vi "Do_ADAM_channel.vi"(4 "Scan Period":dbl format="%.2f", 5 "Previous Scan Value":dbl format="%.2f", 6 "Present scan array":dbl[](array[numeric]) format="%.2f", 7 "Value to Output":dbl format="%.2f", 8 "Ch Description":T1 {"Duty" format="%.0b"; "D" format="%#_5g"; "C" format="%#_5g"; "B" format="%#_5g"; "A" format="%#_5g"}, 9 "Ch names":string[](array[string])) -> (0 "Scan comment":string, 1 "Output":dbl format="%.3f")   [LabVIEW 2011]
uses:
  ADAM Client/Sub VIs/ADAM Controls/Ch_description_ADAM.ctl
  ADAM Client/Sub VIs/ADAM Controls/Module_type_ADAM.ctl
  ADAM Client/Sub VIs/ADAM Controls/Function_ADAM.ctl
  ADAM Client/Sub VIs/ADAM Controls/Channel_State.ctl
  ADAM Client/Sub VIs/ADAM Controls/Calib_type_ADAM.ctl
  ADAM Client/Sub VIs/ADAM Controls/Address.ctl
  ADAM Client/Sub VIs/ADAM Controls/Remember_value_mode.ctl
  ADAM Client/Sub VIs/ADAM Controls/Search_mode.ctl
  Anemometry/Anemometry Sub Vis/Controls/In_Range.ctl
  Anemometry/Anemometry Sub Vis/Globals/Gas_management_global.vi
  ADAM_Global.vi
  Anemometry/Anemometry Sub Vis/Globals/Constants_global.vi
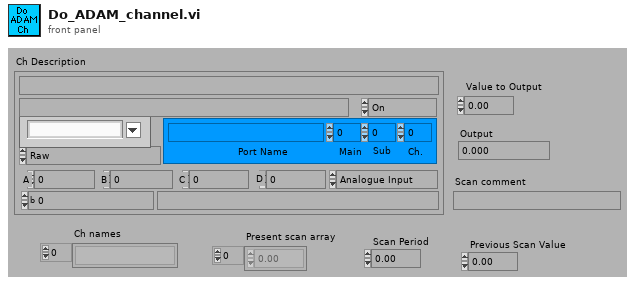
[diagram p1: front panel]
types:
  T1 = typedef "Ch_description_ADAM.ctl" = cluster{"Ch Name":string, "Type":T2, "Function":T3, "Ch State":T4, "Calibration type":T5, "A":dbl, "B":dbl, "C":dbl, "D":dbl, "Comments":string, "Address":T6, "String":string, "Duty":u16}
  T2 = typedef "Module_type_ADAM.ctl" = string
  T3 = typedef "Function_ADAM.ctl" = enum16{"Analogue Input", "Digital Input", "Event counter", "Event rate", "Analogue Output", "Digital Output", "Relay Output"}
  T4 = typedef "Channel_State.ctl" = enum16{"On", "Off", "Always On", "Always Off"}
  T5 = typedef "Calib_type_ADAM.ctl" = enum16{"Raw", "Bx + A", "Cx^2 + Bx + A", "Dx^3 + Cx^2 + Bx + A", "In Band", "Hi-Tec Q", "Hi-Tec M_dot", "Text"}
  T6 = typedef "Address.ctl" = cluster{"Main":i32, "Ch.":i32, "Sub":i32, "Port Name":string}
  T7 = typedef "Remember_value_mode.ctl" = enum16{"Read only", "Read and Write"}
  T8 = typedef "Search_mode.ctl" = enum16{"Between times", "All Times"}
  T9 = typedef "In_Range.ctl" = enum16{"%", "±", "% & ±"}
  T10 = typedef "Valco_valve_ph.ctl" = u16
  T11 = cluster{"Centre Times":dbl[], "Output array":dbl[]}
  T12 = cluster{"Centre Times":dbl[], "Output array":dbl[]}[]
  T13 = typedef "LVDateTimeRec.ctl" = cluster{"fractional second":dbl, "second":i32, "minute":i32, "hour":i32, "day of month":i32, "month":i32, "year":i32, "day of week":i32, "day of year":i32, "DST":i32}
  T14 = typedef "Client_State_Cluster.ctl" = cluster{"Client Name":string, "Traverse level State":T15, "People to Email":string[], "Next Contact Time":dbl}
  T15 = typedef "Traverse_Level_State.ctl" = enum16{"Running", "Complete"}
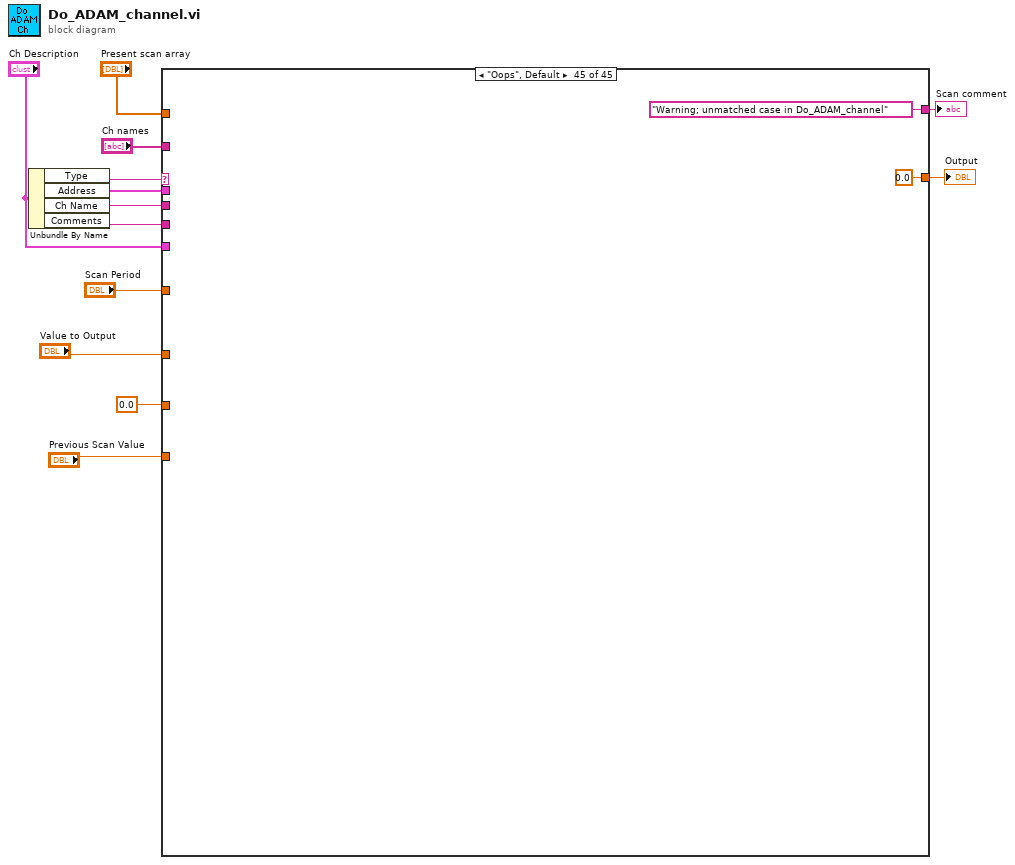
[diagram p0: block diagram]
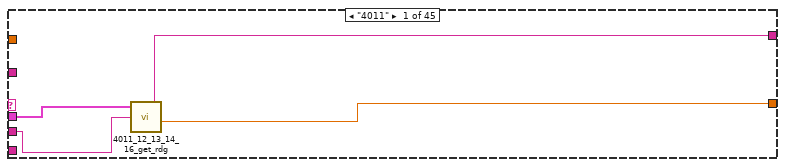
[diagram p2: hidden frame]
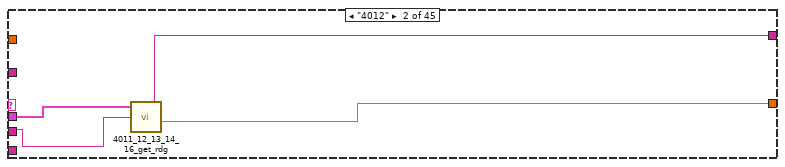
[diagram p3: hidden frame]
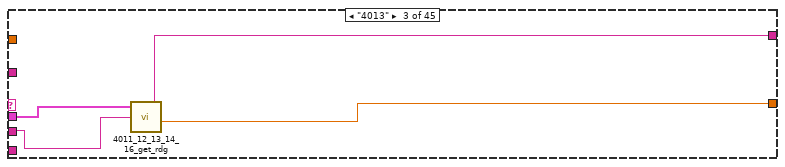
[diagram p4: hidden frame]
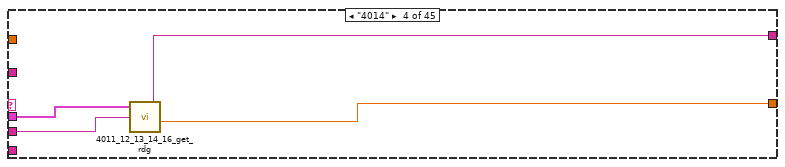
[diagram p5: hidden frame]
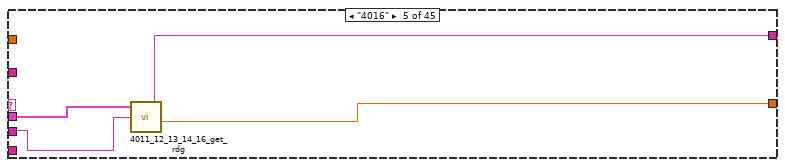
[diagram p6: hidden frame]
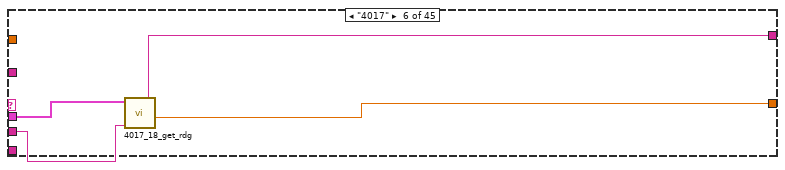
[diagram p7: hidden frame]
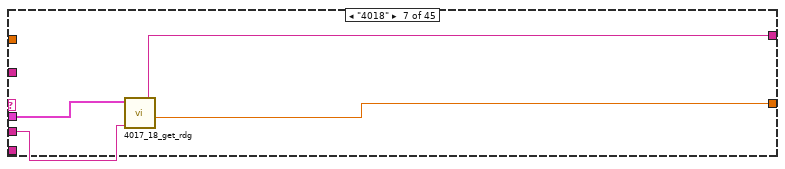
[diagram p8: hidden frame]
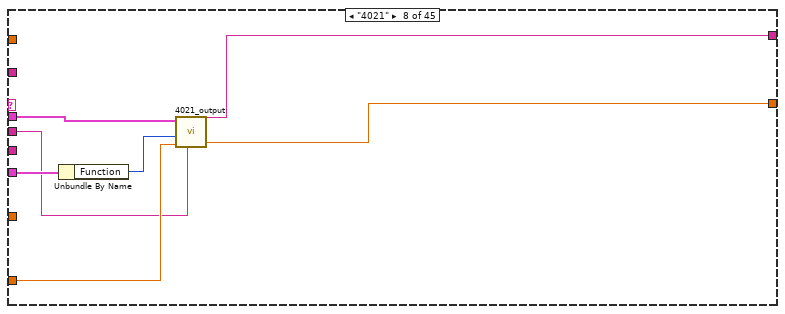
[diagram p9: hidden frame]
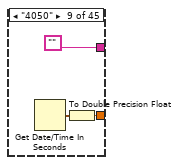
[diagram p10: hidden frame]
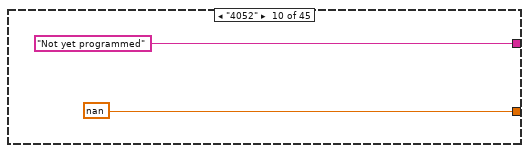
[diagram p11: hidden frame]
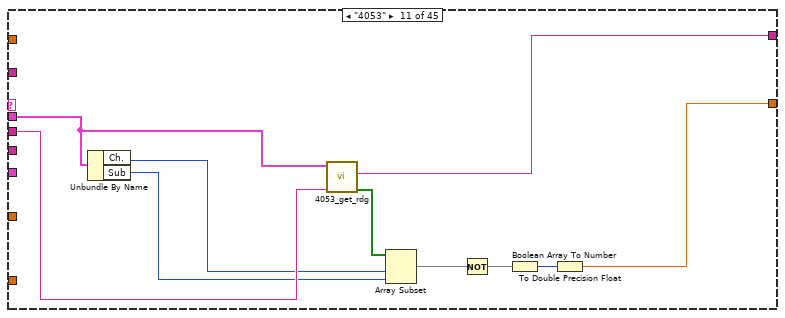
[diagram p12: hidden frame]
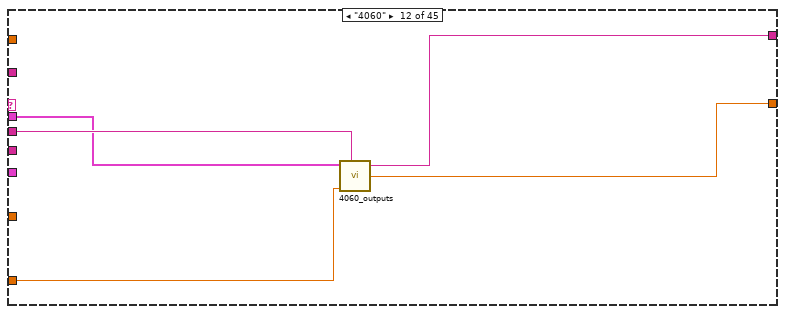
[diagram p13: hidden frame]
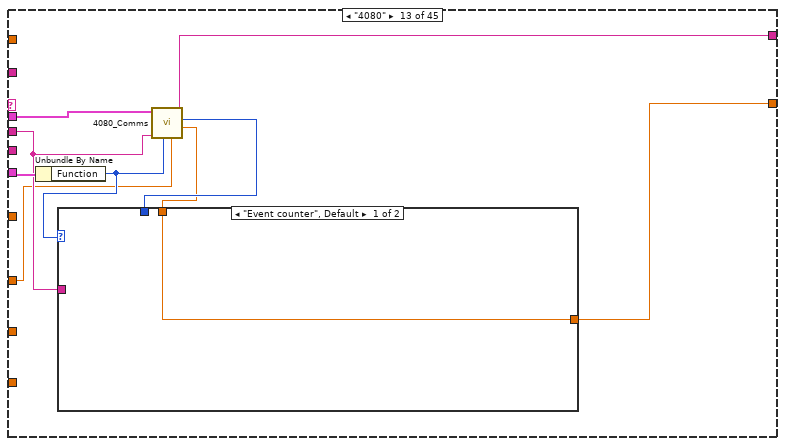
[diagram p14: hidden frame]
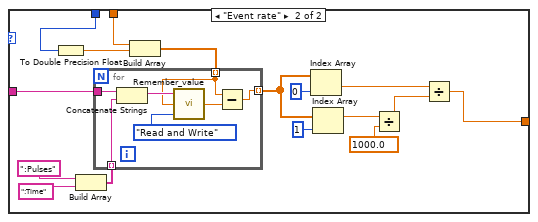
[diagram p15: hidden frame]
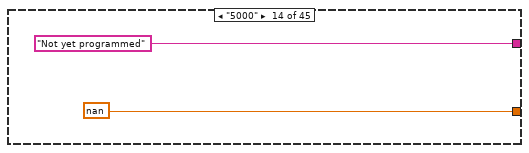
[diagram p16: hidden frame]
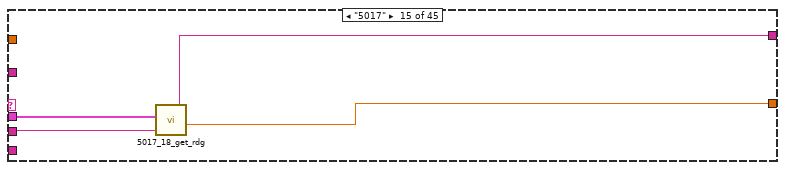
[diagram p17: hidden frame]
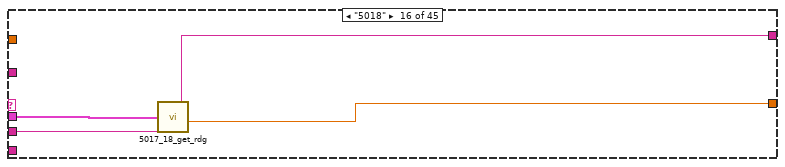
[diagram p18: hidden frame]
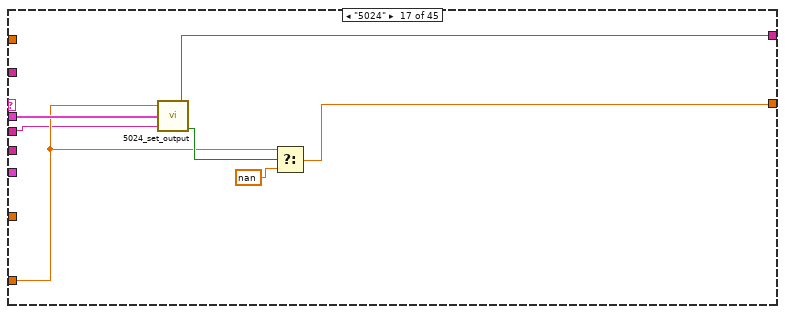
[diagram p19: hidden frame]
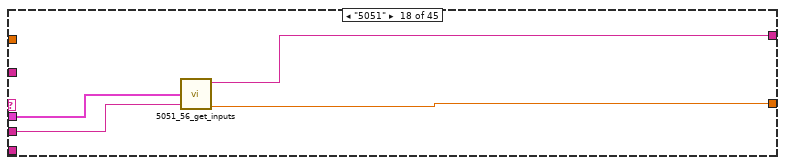
[diagram p20: hidden frame]
diagram:
  n1 = Unbundle By Name("Ch Description") -> ("Type"=w11:T2, "Address"=w10:T6, "Ch Name"=w2:string, "Comments"=w7:string)
  n2 = case shown="\"Oops\", Default" w11 {
    tunnel: [w16 w20 w24 w28 w32 w36 w40 w47 w50 nan w57 w66 w75 nan w105 w109 w114 w120 w128 w149 w171 w190 nan w258 w260 w274 w299 w338 nan w350 w381 w386 w387 w499 w923 w925 w929 w934 w946 w980 w1006 w1016 w1021 w1031 0.0 ("Output")] -> w8
    tunnel: [w17 w21 w25 w29 w33 w37 w41 w48 "" "Not yet programmed" w62 w67 w77 "Not yet programmed" w106 w110 w117 w121 w127 w150 w172 w192 "Not yet programmed" w257 w261 w273 w291 w339 "Not yet programmed" w349 w382 w385 w408 w498 "" "" w930 "" "" w969 "" w1017 w1020 "Crazy time based random number!" "Warning; unmatched case in Do_ADAM_channel" ("Status note")] -> w5
    tunnel: w10 -> [w14 w18 w22 w26 w30 w34 w38 w42 _ _ w54 w65 w69 _ w107 w111 w118 w122 w126 w151 w173 w194 _ w255 w259 w278 w296 w344 _ _ w380 w383 _ w490 _ _ _ _ _ _ w1015 w1019 _ _ _]
    tunnel: "Ch Description" -> [_ _ _ _ _ _ _ w46 _ _ _ _ w76 _ _ _ _ _ w125 w148 w170 w193 _ _ _ _ _ _ _ w355 _ _ w413 w492 _ w926 w931 _ _ _ _ _ w1022 _ _]
    tunnel: w2 -> [w15 w19 w23 w27 w31 w35 w39 w43 _ _ w63 w68 w72 _ w104 w108 w112 w119 w123 w145 w167 w191 _ w256 _ w276 w292 w343 _ _ _ w384 _ w495 _ _ _ _ w942 w976 _ w1018 _ _ _]
    tunnel: "Ch names" -> [_ _ _ _ _ _ _ _ _ _ _ _ _ _ _ _ _ _ _ _ _ _ _ _ _ _ _ _ _ w356 _ _ w412 w497 _ _ w932 _ _ _ _ _ _ _ _]
    tunnel: "Present scan array" -> [_ _ _ _ _ _ _ _ _ _ _ _ _ _ _ _ _ _ _ _ _ _ _ _ _ _ _ _ _ w353 _ _ w410 w496 _ _ w933 _ _ _ _ _ _ _ _]
    tunnel: w7 -> [_ _ _ _ _ _ _ _ _ _ _ _ _ _ _ _ _ _ _ _ _ _ _ _ _ _ _ _ _ w348 _ _ w414 _ _ _ _ _ _ _ _ _ _ _ _]
    tunnel: "Value to Output" -> [_ _ _ _ _ _ _ w44 _ _ _ w64 w70 _ _ _ w113 _ w124 w146 w168 w189 _ _ _ w262 w300 _ _ w354 _ _ _ _ _ _ _ _ _ _ w1010 _ _ _ _]
    tunnel: "Scan Period" -> [_ _ _ _ _ _ _ _ _ _ _ _ _ _ _ _ _ _ _ _ _ _ _ _ _ _ _ _ _ w351 _ _ _ w494 _ _ _ _ _ _ _ _ _ _ _]
    tunnel: "Previous Scan Value" -> [_ _ _ _ _ _ _ _ _ _ _ _ _ _ _ _ _ _ _ _ _ _ _ _ _ _ _ _ _ w352 _ _ w388 w493 w923 _ _ w934 _ _ _ _ _ _ _]
    tunnel: 0.0 -> [_ _ _ _ _ _ _ _ _ _ _ _ _ _ _ _ _ _ _ _ _ _ _ _ _ _ _ _ _ _ _ _ _ w491 _ _ _ _ _ _ _ _ _ _ _]
    frame "4011" {
      n3 = call "4011_12_13_14_16_get_rdg.vi"("Address"=w14, "Channel Name"=w15) -> ("Comment"=w17:string, "Reading"=w16:dbl)  [unwired: 1 in, 2 out]
    }
    frame "4012" {
      n4 = call "4011_12_13_14_16_get_rdg.vi"("Address"=w18, "Channel Name"=w19) -> ("Comment"=w21:string, "Reading"=w20:dbl)  [unwired: 1 in, 2 out]
    }
    frame "4013" {
      n5 = call "4011_12_13_14_16_get_rdg.vi"("Address"=w22, "Channel Name"=w23) -> ("Comment"=w25:string, "Reading"=w24:dbl)  [unwired: 1 in, 2 out]
    }
    frame "4014" {
      n6 = call "4011_12_13_14_16_get_rdg.vi"("Address"=w26, "Channel Name"=w27) -> ("Comment"=w29:string, "Reading"=w28:dbl)  [unwired: 1 in, 2 out]
    }
    frame "4016" {
      n7 = call "4011_12_13_14_16_get_rdg.vi"("Address"=w30, "Channel Name"=w31) -> ("Comment"=w33:string, "Reading"=w32:dbl)  [unwired: 1 in, 2 out]
    }
    frame "4017" {
      n8 = call "4017_18_get_rdg.vi"("Channel Name"=w35, "Address"=w34) -> ("Reading"=w36:dbl, "Comment"=w37:string)  [unwired: 2 in, 2 out]
    }
    frame "4018" {
      n9 = call "4017_18_get_rdg.vi"("Channel Name"=w39, "Address"=w38) -> ("Reading"=w40:dbl, "Comment"=w41:string)  [unwired: 2 in, 2 out]
    }
    frame "4021" {
      n10 = Unbundle By Name(w46) -> ("Function"=w45:T3)
      n11 = call "4021_output.vi"("Address"=w42, "Function"=w45, "Set to:"=w44, "Channel Name"=w43) -> ("Comment"=w48:string, "Reading"=w47:dbl)  [unwired: 1 in, 1 out]
    }
    frame "4050" {
      n12 = Get Date/Time In Seconds() -> (seconds since 1Jan1904=w49:timestamp)
      n13 = To Double Precision Float(number=w49) -> (double precision float=w50:dbl)
    }
    frame "4052" {
    }
    frame "4053" {
      n14 = Unbundle By Name(w54) -> ("Ch."=w55:i32, "Sub"=w61:i32)
      n15 = call "4053_get_rdg.vi"("Channel Name"=w63, "Address"=w54) -> ("Boolean array"=w60:bool[], "Comment"=w62:string)  [unwired: 2 in, 2 out]
      n16 = Array Subset(array=w60, index=w55, length=w61) -> (w59:bool[])
      n17 = Not(x=w59) -> (.not. x?=w56:bool[])
      n18 = Boolean Array To Number(Boolean array=w56) -> (number=w58:u32)
      n19 = To Double Precision Float(number=w58) -> (double precision float=w57:dbl)
    }
    frame "4060" {
      n20 = call "4060_outputs.vi"("Address"=w65, "Value to Output"=w64, "Channel Name"=w68) -> ("Comment"=w67:string, "Reading"=w66:dbl)  [unwired: 2 in, 1 out]
    }
    frame "4080" {
      n21 = Unbundle By Name(w76) -> ("Function"=w71:T3)
      n22 = call "4080_Comms.vi"("Value to display"=w70, "Function"=w71, "Channel Name"=w72, "Address"=w69) -> ("Reading"=w73:dbl, "millisecond timer value"=w74:u32, "Comment"=w77:string)  [unwired: 2 in, 1 out]
      n23 = case shown="\"Event counter\", Default" w71 {
        tunnel: w72 -> [_ w94]
        tunnel: w74 -> [_ w87]
        tunnel: [w78 w79] -> w75
        tunnel: w73 -> [w78 w88]
        frame "Event counter", Default {
        }
        frame "Event rate" {
          n24 = To Double Precision Float(number=w87) -> (double precision float=w86:dbl)
          n25 = Build Array(":Pulses", ":Time") -> (w89:string[])
          n26 = Build Array(w88, w86) -> (w85:dbl[])
          n27 = for {
            tunnel: w94 -> [w98]
            tunnel: [w99] -> w82 mode=indexing
            tunnel: w89 -> [w96] mode=indexing
            tunnel: w85 -> [w95] mode=indexing
            n28 = Concatenate Strings(w98, w96) -> (w97:string)
            n29 = call "Remember_value.vi"("Mode"=Remember_value_mode."Read and Write", "Input Value"=w95, "Ch name"=w97) -> ("Output Value"=w100:dbl)
            n30 = Subtract(x=w95, y=w100) -> (x-y=w99:dbl)
          }
          n31 = Index Array(array=w82, index=0) -> (element=w80:dbl)
          n32 = Index Array(array=w82, index=1) -> (element=w81:dbl)
          n33 = Divide(x=w81, y=1000.0) -> (x/y=w92:dbl)
          n34 = Divide(x=w80, y=w92) -> (x/y=w79:dbl)
        }
      }
    }
    frame "5000" {
    }
    frame "5017" {
      n35 = call "5017_18_get_rdg.vi"("Address (all reqd.)"=w107, "Channel Name"=w104) -> ("Comment"=w106:string, "Reading"=w105:dbl)  [unwired: 3 out]
    }
    frame "5018" {
      n36 = call "5017_18_get_rdg.vi"("Address (all reqd.)"=w111, "Channel Name"=w108) -> ("Comment"=w110:string, "Reading"=w109:dbl)  [unwired: 3 out]
    }
    frame "5024" {
      n37 = call "5024_set_output.vi"("Set to:"=w113, "Address (all reqd.)"=w118, "Channel Name"=w112) -> ("Comment"=w117:string, "Good Reply"=w115:bool)  [unwired: 2 out]
      n38 = Select(t=w113, s=w115, f=nan) -> (s? t:f=w114:dbl)
    }
    frame "5051" {
      n39 = call "5051_56_get_inputs.vi"("Address (Main, Sub reqd.)"=w122, "Channel Name"=w119) -> ("Comment"=w121:string, "Single output"=w120:dbl)  [unwired: 3 out]
    }
    frame "5056" {
      n40 = Unbundle By Name(w125) -> ("Function"=w129:T3)
      n41 = case shown="\"Digital Input\"" w129 {
        tunnel: w126 -> [_ w135 w144]
        tunnel: ["This function is not available" w136 w142] -> w127
        tunnel: [nan ("A") w133 w139] -> w128
        tunnel: w124 -> [_ _ w138]
        tunnel: w123 -> [_ w132 w137]
        frame "Analogue Input", Default {
        }
        frame "Digital Input" {
          # "Readback value"
          n42 = call "5060_check_outputs.vi"("Address (Main, Sub reqd.)"=w135, "Channel Name"=w132) -> ("Comment"=w136:string, "Single Channel"=w134:i16)  [unwired: 3 out]
          n43 = To Double Precision Float(number=w134) -> (double precision float=w133:dbl)
        }
        frame "Relay Output" {
          # "Sets single o/p channel"
          n44 = Greater Than 0?(x=w138) -> (x > 0?=w143:bool)
          n45 = call "5056_60_set_single_output.vi"("Channel Name"=w137, "Address (all reqd.)"=w144, "Set state:"=w143) -> ("Comment"=w142:string, "Good Reply"=w141:bool)  [unwired: 2 out]
          n46 = Select(t=w138, s=w141, f=nan) -> (s? t:f=w139:dbl)
        }
      }
    }
    frame "5060" {
      n47 = Unbundle By Name(w148) -> ("Function"=w147:T3)
      n48 = case shown="\"Relay Output\"" w147 {
        tunnel: w151 -> [_ w157 w166]
        tunnel: ["This function is not available" w158 w164] -> w150
        tunnel: [nan ("A") w155 w161] -> w149
        tunnel: w146 -> [_ _ w160]
        tunnel: w145 -> [_ w154 w159]
        frame "Analogue Input", Default {
        }
        frame "Digital Input" {
          # "Readback value"
          n49 = call "5060_check_outputs.vi"("Address (Main, Sub reqd.)"=w157, "Channel Name"=w154) -> ("Comment"=w158:string, "Single Channel"=w156:i16)  [unwired: 3 out]
          n50 = To Double Precision Float(number=w156) -> (double precision float=w155:dbl)
        }
        frame "Relay Output" {
          # "Sets single o/p channel"
          n51 = Greater Than 0?(x=w160) -> (x > 0?=w165:bool)
          n52 = call "5056_60_set_single_output.vi"("Channel Name"=w159, "Address (all reqd.)"=w166, "Set state:"=w165) -> ("Comment"=w164:string, "Good Reply"=w163:bool)  [unwired: 2 out]
          n53 = Select(t=w160, s=w163, f=nan) -> (s? t:f=w161:dbl)
        }
      }
    }
    frame "6060" {
      n54 = Unbundle By Name(w170) -> ("Function"=w169:T3)
      n55 = case shown="\"Digital Input\"" w169 {
        tunnel: w173 -> [_ w179 w188]
        tunnel: ["This function is not available" w180 w186] -> w172
        tunnel: [nan ("A") w177 w183] -> w171
        tunnel: w168 -> [_ _ w182]
        tunnel: w167 -> [_ w176 w181]
        frame "Analogue Input", Default {
        }
        frame "Digital Input" {
          n56 = call "6060_read_all_I-O.vi"("Address (Main, Sub reqd.)"=w179, "Channel Name"=w176) -> ("Comment"=w180:string, "Single Input Channel"=w178:i16)  [unwired: 3 out]
          n57 = To Double Precision Float(number=w178) -> (double precision float=w177:dbl)
        }
        frame "Relay Output" {
          # "Sets single o/p channel"
          n58 = Greater Than 0?(x=w182) -> (x > 0?=w187:bool)
          n59 = call "6060_set_single_output.vi"("Channel Name"=w181, "Address (Main, Ch requd.)"=w188, "Set state:"=w187) -> ("Comment"=w186:string, "Good Reply"=w185:bool)  [unwired: 2 out]
          n60 = Select(t=w182, s=w185, f=nan) -> (s? t:f=w183:dbl)
        }
      }
    }
    frame "Tracker" {
      n61 = while {
        tunnel: w194 -> [w218]
        tunnel: w193 -> [w217]
        tunnel: [w211] -> w192
        tunnel: w191 -> [w210]
        tunnel: [w204] -> w190
        tunnel: w189 -> [w203]
        i -> [w200]
        stop <- w197 continue-if-true
        n62 = Unbundle By Name(w217) -> ("Function"=w216:T3)
        n63 = Unbundle By Name(w218) -> ("Port Name"=w215:string, "Ch."=w206:i32, "Main"=w214:i32, "Sub"=w213:i32)
        n64 = case shown="\"Analogue Output\"" w216 {
          tunnel: [enum16{"Set", "Read"}."Set" ("Set") enum16{"Set", "Read"}."Set" ("Set") enum16{"Set", "Read"}."Set" ("Set") enum16{"Set", "Read"}."Set" ("Set") enum16{"Set", "Read"}."Set" ("Set") enum16{"Set", "Read"}."Read" ("Set") enum16{"Set", "Read"}."Read" ("Set")] -> w201
          tunnel: [enum16{"Logic", "Analogue"}."Analogue" ("Analogue") enum16{"Logic", "Analogue"}."Logic" ("Analogue") enum16{"Logic", "Analogue"}."Logic" ("Analogue") enum16{"Logic", "Analogue"}."Logic" ("Analogue") enum16{"Logic", "Analogue"}."Logic" ("Analogue") enum16{"Logic", "Analogue"}."Logic" ("Analogue") enum16{"Logic", "Analogue"}."Analogue" ("Analogue")] -> w212
          frame "Analogue Output" {
          }
          frame "Digital Output" {
          }
          frame "Relay Output" {
          }
          frame "Event rate" {
          }
          frame "Event counter" {
          }
          frame "Digital Input" {
          }
          frame "Analogue Input" {
          }
        }
        n65 = call "TalkTracker.vi"("PORT NAME"=w215, "Set"=w201, "Channel Name"=w210, "Value to set"=w203, "MODULE ADDRESS"=w214, "LOCATION"=w206, "NO. LOCATIONS"=w213, "Analogue"=w212) -> ("Response"=w208:string, "Good Set?"=w195:bool, "Comment out"=w211:string)  [unwired: 1 in, 4 out]
        n66 = Match Pattern(string=w208, regular expression="\r\n") -> (before substring=w207:string)  [unwired: 4 out]
        n67 = case shown="\"Set\"" w201 {
          tunnel: w207 -> [_ w230]
          tunnel: [w222 w229] -> w205
          tunnel: w203 -> [w224 _]
          tunnel: nan ("Reading") -> [w223 w228]
          tunnel: [w221 w226] -> w198
          tunnel: [0 ("y") 1 ("y")] -> w196
          tunnel: w195 -> [w219 _]
          frame "Set" {
            n68 = Not(x=w219) -> (.not. x?=w221:bool)
            n69 = Select(t=w224, s=w219, f=w223) -> (s? t:f=w222:dbl)
          }
          frame "Read" {
            n70 = String Length(string=w230) -> (length=w232:i32)
            n71 = Fract/Exp String To Number(string=w230, default (0 dbl)=w228) -> (offset past number=w233:i32, number=w231:dbl)  [unwired: 2 out]
            n72 = Equal?(x=w232, y=w233) -> (x = y?=w227:bool)
            n73 = Not(x=w227) -> (.not. x?=w226:bool)
            n74 = Select(t=w231, s=w227, f=w228) -> (s? t:f=w229:dbl)
          }
        }
        n75 = case shown="0, Default" w206 {
          tunnel: w205 -> [w234 w237]
          tunnel: [w234 w235] -> w204
          frame 0, Default {
          }
          frame 283 {
            n76 = Equal To 0?(x=w237) -> (x = 0?=w238:bool)
            n77 = Select(t=nan ("Reading"), s=w238, f=w237) -> (s? t:f=w235:dbl)
          }
        }
        n78 = Less?(x=w200, y=w196) -> (x < y?=w199:bool)
        n79 = And(x=w198, y=w199) -> (x .and. y?=w197:bool)
      }
    }
    frame "WEST" {
    }
    frame "GILL" {
      n80 = call "Gill_get_rdg.vi"("Channel Name"=w256, "Address"=w255) -> ("Output"=w258:dbl, "Status note"=w257:string)  [unwired: 2 in, 2 out]
    }
    frame "ClimatronicsUDP" {
      n81 = call "ClimatronicsUDP_get_rdg.vi"("Address"=w259) -> ("Output"=w260:dbl, "Status note"=w261:string)  [unwired: 5 in]
    }
    frame "JEM" {
      n82 = Unbundle By Name(w278) -> ("Main"=w265:i32, "Ch."=w264:i32, "Port Name"=w277:string)
      n83 = case shown="0, Default" w264 {
        tunnel: [i16[] [-3, -2, -1, 0, 14, 29, 43, 57, 71, 86, 100] i16[] [0, 20, 40, 60, 80, 100, 120]] -> w268
        tunnel: [u8[] [10, 50, 80, 100, 120, 140, 160, 180, 200, 220, 240] u8[] [20, 50, 90, 130, 160, 200, 230]] -> w269
        frame 0, Default {
        }
        frame 1 {
        }
      }
      n84 = Add(x=w265, y=w264) -> (x+y=w263:i32)
      n85 = Threshold 1D Array(2:w262, 3:w268) -> (0:w271:dbl)  [unwired: 1 out]
      n86 = Round To Nearest(number=w271) -> (nearest integer value=w272:dbl)
      n87 = To Long Integer(number=w272) -> (32bit integer=w270:i32)
      n88 = Index Array(array=w269, index=w270) -> (element=w267:u8)
      n89 = call "DMX.vi"("Port Name"=w277, "DMX channel no."=w263, "Set value:"=w267, "Channel Name"=w276) -> ("error"=w275:bool)  [unwired: 2 out]
      n90 = Index Array(array=w268, index=w270) -> (element=w266:i16)
      n91 = case shown="False" w275 {
        tunnel: [w279 nan] -> w274
        tunnel: ["" "Comms Error"] -> w273
        tunnel: w266 -> [w281 _]
        frame False {
          n92 = To Double Precision Float(number=w281) -> (double precision float=w279:dbl)
        }
        frame True {
        }
      }
    }
    frame "VICI" {
      n93 = To Long Integer(number=w300) -> (32bit integer=w295:i32)
      n94 = Unbundle By Name(w296) -> ("Port Name"=w298:string, "Ch."=w297:i32)
      n95 = call "Valco_Valve_Position.vi"("Channel Name"=w292, "Valve Number"=w297, "Port Name"=w298, "Requested Posn."=w295) -> ("Error Message"=w290:string, "Achieved Posn."=w293:T10)  [unwired: 2 out]
      n96 = Empty String/Path?(string/path=w290) -> ()  [unwired: 1 out]
      n97 = case shown="True" TRUE {
        tunnel: w296 -> [w307 _]
        tunnel: w295 -> [w306 _]
        tunnel: [w305 w337] -> w294
        tunnel: w293 -> [_ w337]
        tunnel: w292 -> [w304 _]
        tunnel: [w303 w336] -> w291
        tunnel: w290 -> [_ w336]
        tunnel: w290 -> [w302 _]
        tunnel: "X10" ("Port Name") -> [w301 _]
        frame False {
          n98 = stacked-sequence {
            tunnel: w307 -> [_ _ _ _ _ w328]
            tunnel: w306 -> [_ _ _ _ _ w324]
            tunnel: [_ _ _ _ _ w327] -> w305
            tunnel: w304 -> [_ _ _ _ _ w326]
            tunnel: [_ _ _ _ _ w325] -> w303
            tunnel: w302 -> [_ w313 _ _ _ _]
            tunnel: w301 -> [w308 _ _ w316 _ _]
            frame #0 {
              w310 = 3 items=["-----", "A", "B", "C", "D", "E", "F", "G", "H", "I", "J", "K", "L", "M", "N", "O", "P"] ("House Code")
              n99 = call "X10control.vi"("Port Name"=w308, "Power Request (ON)"=FALSE, "House Code"=w310, "Unit No."=5) -> ()  [unwired: 6 out]
            }
            frame #1 {
              n100 = call "Server_Emails.vi"("Message"=w313, "Contact All clients?"=TRUE, "Subject"="Powering Down FID Valve" ("Error Type")) -> ()  [unwired: 2 in, 3 out]
            }
            frame #2 {
              n101 = Wait (ms)(milliseconds to wait=u32 20000) -> ()  [unwired: 1 out]
            }
            frame #3 {
              w318 = 3 items=["-----", "A", "B", "C", "D", "E", "F", "G", "H", "I", "J", "K", "L", "M", "N", "O", "P"] ("House Code")
              n102 = call "X10control.vi"("Port Name"=w316, "Power Request (ON)"=TRUE, "House Code"=w318, "Unit No."=5) -> ()  [unwired: 6 out]
            }
            frame #4 {
              n103 = Wait (ms)(milliseconds to wait=u32 5000) -> ()  [unwired: 1 out]
            }
            frame #5 {
              n104 = Build Array(1 ("element"), 2 ("element"), w324) -> (w321:i32[])
              n105 = for {
                tunnel: w328 -> [w333]
                tunnel: [w332] -> w327
                tunnel: w326 -> [w331]
                tunnel: [w330] -> w325
                tunnel: w321 -> [w329] mode=indexing
                n106 = Unbundle By Name(w333) -> ("Port Name"=w334:string, "Ch."=w335:i32)
                n107 = call "Valco_Valve_Position.vi"("Channel Name"=w331, "Valve Number"=w335, "Port Name"=w334, "Requested Posn."=w329) -> ("Error Message"=w330:string, "Achieved Posn."=w332:T10)  [unwired: 2 out]
              }
            }
          }
        }
        frame True {
        }
      }
      n108 = To Double Precision Float(number=w294) -> (double precision float=w299:dbl)
    }
    frame "Vaisala" {
      n109 = Unbundle By Name(w344) -> ("Main"=w340:i32, "Ch."=w341:i32, "Port Name"=w342:string)
      n110 = call "HMP231.vi"("Channel Name"=w343, "Port Name"=w342, "Channel"=w341, "Address"=w340) -> ("Output"=w338:dbl, "Status note"=w339:string)  [unwired: 2 out]
    }
    frame "DRUCK" {
    }
    frame "Run VI Named:" {
      n111 = Current VI's Path() -> (path=w365:path)
      n112 = Strip Path(path=w365) -> (stripped path=w366:path)  [unwired: 1 out]
      n113 = call <vilib>:"Trim Whitespace.vi"("string"=w348) -> ("trimmed string"=w347:string)  [unwired: 1 in]
      n114 = Strip Path(path=w366) -> (stripped path=w367:path)  [unwired: 1 out]
      n115 = Build Path(base path=w367, name or relative path="Run_vi_named") -> (appended path=w369:path)
      n116 = Build Path(base path=w369, name or relative path=w347) -> (appended path=w364:path)
      n117 = Open VI Reference(type specifier VI Refnum (for type only)=refnum<vi> refnum, vi path=w364) -> (vi reference=w360:refnum<vi>, error out=w359:errorcluster)  [unwired: 1 in, 3 out]
      n118 = property class="VI Interface Type 7"(reference=w360, error in=w359) -> (reference out=w362:refnum<vi>, error out=w361:errorcluster, "Front Panel Window:Open"=w363:bool)
      n119 = case shown="False" w363 {
        tunnel: w362 -> [w377 w379]
        tunnel: w361 -> [w376 w378]
        tunnel: [w375 w379] -> w358
        tunnel: [w373 w378] -> w357
        frame False {
          n120 = property class="VI Interface Type 7"(reference=w377, error in=w376, "Front Panel Window:Open"=TRUE) -> (reference out=w375:refnum<vi>, error out=w373:errorcluster)
        }
        frame True {
        }
      }
      n121 = call-by-ref "?"(reference=w358, error in=w357, "Scan Period"=w351, "Previous Scan Value"=w352, "Present scan array"=w353, "Value to Output"=w354, "Ch Description"=w355, "Ch names"=w356) -> (reference out=w371:refnum<vi>, error out=w372:errorcluster, "Scan comment"=w349:string, "Output"=w350:dbl)  [unwired: 2 in]
      n122 = Close Reference(reference=w371, error in (no error)=w372) -> ()  [unwired: 1 out]
    }
    frame "IR2100" {
      n123 = call "IR2100_get_rdg.vi"("Address"=w380) -> ("Comment"=w382:string, "Reading"=w381:dbl)  [unwired: 2 in, 2 out]
    }
    frame "PPT" {
      n124 = call "PPT_get_rdg.vi"("Channel Name"=w384, "Address"=w383) -> ("Reading"=w386:dbl, "Comment"=w385:string)  [unwired: 2 in, 2 out]
    }
    frame "Comparator" {
      # "A Warn if above this value\nB Warn if below this value\nC  Hysteresis margin\nD is the averaging time in minutes\nComments   is Channel name to check"
      n125 = Unbundle By Name(w413) -> ("D"=w396:dbl)
      n126 = Match Pattern(string=w414, regular expression=":::" ("String to match")) -> (before substring=w411:string)  [unwired: 4 out]
      n127 = call "Read_value_of_earlier_Ch.vi"("Desired Ch to Read"=w411, "Ch names"=w412, "Present scan array"=w410) -> ("Value"=w395:dbl, "Scan comment"=w409:string)  [unwired: 1 in]
      n128 = Equal?(x=w388, y=1.0) -> (x = y?=w404:bool)
      n129 = Unbundle By Name(w413) -> ("A"=w407:dbl, "B"=w406:dbl, "C"=w405:dbl)
      n130 = Equal To 0?(x=w396) -> (x = 0?=w394:bool)
      n131 = case shown="True" w404 {
        tunnel: [w420 w425] -> w402
        tunnel: w407 -> [w420 w424]
        tunnel: w406 -> [w419 w423]
        tunnel: [w419 w421] -> w403
        tunnel: w405 -> [_ w422]
        frame False {
        }
        frame True {
          n132 = Subtract(x=w424, y=w422) -> (x-y=w425:dbl)
          n133 = Add(x=w423, y=w422) -> (x+y=w421:dbl)
        }
      }
      n134 = case shown="False" w394 {
        tunnel: [w430 w433] -> w417
        tunnel: w411 -> [w432 _]
        tunnel: [w428 w434] -> w393
        tunnel: w396 -> [w426 _]
        tunnel: w395 -> [_ w434]
        tunnel: w409 -> [w430 w433]
        frame False {
          n135 = Build Array(w432) -> (w427:string[])
          n136 = call "Get_Channel_averages.vi"("Desired Ch Names"=w427, "Averaging time (mins)"=w426) -> ("number"=w429:dbl[])  [unwired: 1 in, 2 out]
          n137 = Index Array(array=w429, index=0) -> (element=w428:dbl)
        }
        frame True {
        }
      }
      n138 = Not(x=w404) -> (.not. x?=w397:bool)
      n139 = In Range and Coerce(upper limit=w402, x=w393, lower limit=w403) -> (In Range?=w398:bool)  [unwired: 1 out]
      n140 = Greater?(x=w393, y=w402) -> (0:w401:bool)
      n141 = Not A Number/Path/Refnum?(number/path/refnum=w393) -> (NaN/Path/Refnum?=w390:bool)
      n142 = Equal?(x=w398, y=w397) -> (x = y?=w392:bool)
      n143 = Or(x=w392, y=w390) -> (x .or. y?=w391:bool)
      n144 = case shown="False" w391 {
        tunnel: w411 -> [w441 _]
        tunnel: w402 -> [w440 _]
        tunnel: w413 -> [w439 _]
        tunnel: w403 -> [w438 _]
        tunnel: w398 -> [w437 _]
        tunnel: w393 -> [w436 _]
        tunnel: w401 -> [w435 _]
        frame False {
          n145 = stacked-sequence {
            seq-local: [w447 _ _ _ _] -> [_ _ _ w488 _]
            seq-local: [_ w467 _ _ _] -> [_ _ _ w485 _]
            seq-local: [w445 _ _ _ _] -> [_ _ _ w481 _]
            tunnel: w441 -> [w449 w475 _ w487 _]
            tunnel: w440 -> [w448 _ _ _ _]
            tunnel: w439 -> [_ _ w480 w489 _]
            tunnel: w438 -> [w446 _ _ _ _]
            tunnel: w437 -> [w444 _ _ _ _]
            tunnel: w436 -> [w443 _ _ _ _]
            tunnel: w435 -> [w442 _ _ _ _]
            frame #0 {
              n146 = case shown="True" w444 {
                tunnel: w449 -> [w454 w465]
                tunnel: w448 -> [_ w458]
                tunnel: [w452 w464] -> w447
                tunnel: w446 -> [_ w457]
                tunnel: ["OK " ""] -> w445
                tunnel: w443 -> [w450 _]
                tunnel: w442 -> [_ w455]
                frame True {
                  n147 = Format Into String(format string="The channel named %s is now  %.3f" ("Format String"), w454, w450) -> (resulting string=w452:string)  [unwired: 2 in, 1 out]
                }
                frame False {
                  n148 = Select(t=w458, s=w455, f=w457) -> (s? t:f=w456:dbl)
                  n149 = Select(t="greater", s=w455, f="less") -> (s? t:f=w460:string)
                  n150 = Format Into String(format string="%s is %s than %.3f" ("Format String"), w465, w460, w456) -> (resulting string=w464:string)  [unwired: 2 in, 1 out]
                }
              }
            }
            frame #1 {
              n151 = Build Array(w475) -> (w474:string[])
              n152 = call "Channel_Names_and_indicies.vi"("All Active Channels"=FALSE, "Desired Ch Names"=w474) -> ("Indicies"=w472:i32[])  [unwired: 1 out]
              n153 = call "Specified_Channels_server.vi"("Mode"=Search_mode."All Times", "Requested channels"=w472) -> ("Output array"=w470:dbl[][], "Centre Times"=w466:dbl[])  [unwired: 3 in, 3 out]
              n154 = Index Array(array=w470, index (row)=0) -> (element=w468:dbl[])  [unwired: 1 in]
              n155 = Bundle("Centre Times"=w466, "Output array"=w468) -> (w471:T11)  [unwired: 1 out]
              n156 = Build Array(w471) -> (w467:T12)
            }
            frame #2 {
              w478 = TRUE  # Contact All clients?
              n157 = Unbundle By Name(w480) -> ("String"=w479:string)
              n158 = call "Get_array_values_fr_String.vi"("String Value"=w479) -> ("String array"=w477:string[])  [unwired: 1 out]
              n159 = call "Client_email_addresses.vi"("Extra People to Email"=w477, "Contact All clients?"=w478) -> ()  [unwired: 1 in]
            }
            frame #3 {
              n160 = Unbundle By Name(w489) -> ("Ch Name"=w482:string)
              n161 = Build Array(w487) -> (w486:string[])
              n162 = Concatenate Strings(w481, w482) -> (w483:string)
              n163 = call "Email_Attachment_Plot.vi"("X axis name"="Time", "XY Graph"=w485, "Series Names"=w486, "message"=w488, "subject ([No Subject])"=w483) -> ()  [unwired: 1 in, 1 out]
            }
            frame #4 {
            }
          }
        }
        frame True {
        }
      }
      n164 = Concatenate Strings(w417, "") -> (w408:string)
      n165 = Select(t=0.0, s=w398, f=1.0) -> (s? t:f=w389:dbl)
      n166 = Select(t=w388, s=w390, f=w389) -> (s? t:f=w387:dbl)
    }
    frame "VIRTUAL" {
      n167 = case shown="\"Laser:Cooling_Water:Delta_T\"" w495 {
        tunnel: [w509 w523 w537 w559 w574 w585 w601 w632 w659 w694 w703 w720 w773 w799 w826 w846] -> w499
        tunnel: [w500 w529 w535 w563 w568 w583 w610 "" w663 w688 w697 w717 w772 w798 "" w847] -> w498
        tunnel: w497 -> [w506 w531 w541 w565 w570 w588 w612 w636 w665 w690 w699 w718 w778 w803 _ w849]
        tunnel: w496 -> [w507 w530 w542 w564 w569 w589 w611 w637 w666 w689 w698 w719 w780 w805 _ w848]
        tunnel: w495 -> [w504 _ _ _ _ _ _ _ _ _ _ w706 _ _ w821 _]
        tunnel: w494 -> [w505 _ _ _ _ _ _ _ _ _ _ _ w770 w797 w826 w845]
        tunnel: w493 -> [w508 _ _ _ _ _ _ _ _ _ _ w721 w774 w800 _ w844]
        tunnel: w492 -> [_ _ w533 _ _ _ _ _ _ _ _ w712 _ _ _ _]
        tunnel: w491 -> [_ w522 _ _ _ w582 _ _ _ _ _ _ _ _ _ _]
        tunnel: w490 -> [_ _ _ _ _ _ _ _ _ _ _ _ _ _ _ _]
        frame "GMU:Remaining:", Default {
          n168 = Match Pattern(string=w504, regular expression="GMU:Remaining:" ("String to match")) -> (match substring=w502:string)  [unwired: 4 out]
          n169 = Empty String/Path?(string/path=w502) -> (empty?=w501:bool)
          n170 = case shown="False" w501 {
            tunnel: [w516 nan] -> w509
            tunnel: w508 -> [w515 _]
            tunnel: w507 -> [w514 _]
            tunnel: w506 -> [w513 _]
            tunnel: w505 -> [w512 _]
            tunnel: w504 -> [w511 _]
            tunnel: [w510 w518] -> w500
            frame False {
              n171 = call "Update_Rem_gas.vi"("Scan Period (s)"=w512, "Gas Remaining in"=w515, "Ch name"=w511, "Ch names"=w513, "Present scan array"=w514) -> ("Gas Remaining out"=w516:dbl, "Comments"=w510:string)  [unwired: 1 out]
            }
            frame True {
              n172 = Current VI's Path() -> (path=w520:path)
              n173 = Path To String(path=w520) -> (string=w519:string)
              n174 = Concatenate Strings(" was not matched in ", w519) -> (w518:string)
            }
          }
        }
        frame "GMU:Source:Meas Q" {
          n175 = call "Calculate_Release_Flowrates.vi"("Ch names"=w531, "Units"=enum16{"Q l/min", "M_dot Kg/min"}."Q l/min", "Present scan array"=w530) -> ("Trace"=w527:dbl, "Carrier"=w528:dbl, "Scan comments"=w529:string)
          n176 = Add(x=w528, y=w527) -> (x+y=w524:dbl)
          n177 = Not Equal To 0?(x=w524) -> (x != 0?=w525:bool)
          n178 = Select(t=w524, s=w525, f=w522) -> (s? t:f=w523:dbl)
        }
        frame "GMU:Detector:Strength" {
          n179 = Unbundle By Name(w533) -> ("C"=w532:dbl)
          n180 = call "Read_value_of_earlier_Ch.vi"("Desired Ch to Read"="GMU:Detector:Meas Current", "Ch names"=w541, "Present scan array"=w542) -> ("Value"=w538:dbl, "Scan comment"=w536:string)  [unwired: 1 in]
          n181 = Greater?(x=w538, y=w532) -> (0:w539:bool)
          n182 = case shown="True" w539 {
            tunnel: w533 -> [_ w554]
            tunnel: w538 -> [_ w549]
            tunnel: [100.0 ("Eng Values") w547] -> w537
            tunnel: ["Fault" w550] -> w534
            frame False {
            }
            frame True {
              n183 = Unbundle By Name(w554) -> ("D"=w545:dbl, "A"=w553:dbl, "B"=w552:dbl)
              n184 = Less?(x=w549, y=w545) -> (x < y?=w548:bool)
              n185 = Build Array(w553, w552) -> (w551:dbl[])
              n186 = call "Polynomial_convert.vi"("Calib constants"=w551, "Voltage"=w549) -> ("Eng Values"=w546:dbl)  [unwired: 4 out]
              n187 = case shown="True" w548 {
                tunnel: ["Saturated" ""] -> w550
                tunnel: [100.0 ("Eng Values") w557] -> w547
                tunnel: w546 -> [_ w557]
                frame False {
                }
                frame True {
                }
              }
            }
          }
          n188 = Concatenate Strings(w536, w534) -> (w535:string)
        }
        frame "GMU:Source:Meas M_dot" {
          n189 = call "Calculate_Release_Flowrates.vi"("Ch names"=w565, "Units"=enum16{"Q l/min", "M_dot Kg/min"}."M_dot Kg/min", "Present scan array"=w564) -> ("Trace"=w561:dbl, "Carrier"=w562:dbl, "Scan comments"=w563:string)
          n190 = Add(x=w562, y=w561) -> (x+y=w559:dbl)
        }
        frame "GMU:Source:Meas Density" {
          n191 = Build Array("GMU:Source:Meas M_dot", "GMU:Source:Meas Q") -> (w571:string[])
          n192 = call "Read_Earlier_Channels.vi"("Present scan array"=w569, "Ch names"=w570, "Desired Channels"=w571) -> ("Scan comments"=w568:string, "Index 0"=w567:dbl, "Index 1"=w566:dbl)  [unwired: 3 out]
          n193 = Not Equal To 0?(x=w567) -> (x != 0?=w575:bool)
          n194 = case shown="False" w575 {
            tunnel: w567 -> [_ w579]
            tunnel: w566 -> [_ w578]
            tunnel: [0.0 w577] -> w574
            frame False {
            }
            frame True {
              n195 = Divide(x=w579, y=w578) -> (x/y=w580:dbl)
              n196 = Multiply(x=w580, y=1000.0) -> (x*y=w577:dbl)
            }
          }
        }
        frame "GMU:Source:Meas Den Ratio" {
          n197 = call "Read_value_of_earlier_Ch.vi"("Desired Ch to Read"="GMU:Source:Meas Density", "Ch names"=w588, "Present scan array"=w589) -> ("Value"=w584:dbl, "Scan comment"=w583:string)  [unwired: 1 in]
          n198 = Equal?(x=w584, y=w582) -> (x = y?=w586:bool)
          n199 = case shown="False" w586 {
            tunnel: w584 -> [w591 _]
            tunnel: [w590 w596] -> w585
            tunnel: w582 -> [_ w596]
            frame False {
              n200 = global read "Gas_management_global.vi" "Release temp (deg C)"() -> (w594:dbl)
              n201 = global read "Gas_management_global.vi" "Atmos Pres (mbars)"() -> (w593:dbl)
              n202 = call "Gas_Density.vi"("Pressure (mbars)"=w593, "Temperature (deg C)"=w594, "Gas Name"="Air") -> ("Density Kg/m3"=w592:dbl)
              n203 = Divide(x=w591, y=w592) -> (x/y=w590:dbl)
            }
            frame True {
            }
          }
        }
        frame "GMU:Source:Meas Strength" {
          n204 = call "Calculate_Release_Flowrates.vi"("Ch names"=w612, "Units"=enum16{"Q l/min", "M_dot Kg/min"}."Q l/min", "Present scan array"=w611) -> ("Trace"=w604:dbl, "Carrier"=w605:dbl, "Scan comments"=w610:string)
          n205 = Equal To 0?(x=w605) -> (x = 0?=w607:bool)
          n206 = Equal To 0?(x=w604) -> (x = 0?=w608:bool)
          n207 = And(x=w607, y=w608) -> (x .and. y?=w606:bool)
          n208 = case shown="False" w606 {
            tunnel: w605 -> [w623 _]
            tunnel: w604 -> [w622 _]
            tunnel: [w621 0.0] -> w600
            frame False {
              n209 = Add(x=w623, y=w622) -> (x+y=w626:dbl)
              n210 = Divide(x=w622, y=w626) -> (x/y=w625:dbl)
              n211 = Multiply(x=w625, y=100.0) -> (x*y=w621:dbl)
            }
            frame True {
            }
          }
          n212 = while {
            tunnel: [w614] -> w597
            tunnel: [w615] -> w599
            tunnel: w600 -> [w620]
            shift-left: _ -> [w614]
            shift-left: _ -> [w619]
            shift-right: [w620] -> _
            stop <- FALSE continue-if-true
            w618 = 6.0 ("y")
            n213 = Less?(x=w619, y=w618) -> (x < y?=w617:bool)
            n214 = Less?(x=w614, y=w618) -> (x < y?=w616:bool)
            n215 = Or(x=w617, y=w616) -> (x .or. y?=w615:bool)
          }
          n216 = Greater?(x=w600, y=7.0) -> (0:w598:bool)
          n217 = And(x=w599, y=w598) -> (x .and. y?=w602:bool)
          n218 = Select(t=w597, s=w602, f=w600) -> (s? t:f=w601:dbl)
        }
        frame "EnFlo_Tunnel:Temp:Inlet_Av" {
          w635 = 0.0 ("Value")
          w629 = "EnFlo_Tunnel:Temp:Inlet"
          n219 = String Length(string=w629) -> (length=w630:i32)
          n220 = for {
            tunnel: w637 -> [w643] mode=indexing
            tunnel: w636 -> [w642] mode=indexing
            shift-right: [w650] -> w634
            shift-left: w635 -> [w649]
            shift-right: [w647] -> w633
            shift-left: w635 -> [w648]
            tunnel: w630 -> [w646]
            tunnel: w629 -> [w644]
            tunnel: "EnFlo_Tunnel:Temp:Inlet_Av" -> [w641]
            n221 = String Subset(string=w642, length (rest)=w646) -> (substring=w645:string)  [unwired: 1 out]
            n222 = Equal?(x=w645, y=w644) -> (x = y?=w639:bool)
            n223 = Not Equal?(x=w642, y=w641) -> (x != y?=w640:bool)
            n224 = And(x=w639, y=w640) -> (x .and. y?=w638:bool)
            n225 = case shown="True" w638 {
              tunnel: [w652 w656] -> w650
              tunnel: w649 -> [w652 w657]
              tunnel: w643 -> [_ w655]
              tunnel: w648 -> [w651 w654]
              tunnel: [w651 w653] -> w647
              frame False {
              }
              frame True {
                n226 = Add(x=w655, y=w657) -> (x+y=w656:dbl)
                n227 = Increment(x=w654) -> (x+1=w653:dbl)
              }
            }
          }
          n228 = Divide(x=w634, y=w633) -> (x/y=w632:dbl)
        }
        frame "EnFlo Lab:labstrat1:Av Temp" {
          w662 = 0.0 ("Value")
          n229 = for {
            tunnel: w666 -> [w678]
            tunnel: w665 -> [w677]
            shift-right: [w674] -> w663
            shift-left: "" -> [w675]
            shift-right: [w672] -> w661
            shift-left: w662 -> [w671]
            shift-right: [w668] -> w660
            shift-left: w662 -> [w669]
            tunnel: string[] ["EnFlo Lab:labstrat1:Z=4.5m", "EnFlo Lab:labstrat1:Z=3.5m", "EnFlo Lab:labstrat1:Z=2.5m", "EnFlo Lab:labstrat1:Z=1.5m", "EnFlo Lab:labstrat1:Z=0.5m"] -> [w667] mode=indexing
            n230 = call "Read_value_of_earlier_Ch.vi"("Desired Ch to Read"=w667, "Ch names"=w677, "Present scan array"=w678) -> ("Value"=w670:dbl, "Scan comment"=w676:string)  [unwired: 1 in]
            n231 = Concatenate Strings(w675, w676) -> (w674:string)
            n232 = Not A Number/Path/Refnum?(number/path/refnum=w670) -> (NaN/Path/Refnum?=w673:bool)
            n233 = case shown="True" w673 {
              tunnel: [w682 w685] -> w672
              tunnel: w671 -> [w683 w685]
              tunnel: w670 -> [w681 _]
              tunnel: w669 -> [w680 w684]
              tunnel: [w679 w684] -> w668
              frame False {
                n234 = Add(x=w681, y=w683) -> (x+y=w682:dbl)
                n235 = Increment(x=w680) -> (x+1=w679:dbl)
              }
              frame True {
              }
            }
          }
          n236 = Divide(x=w661, y=w660) -> (x/y=w659:dbl)
        }
        frame "EnFlo Lab:labstrat1:Delta T" {
          n237 = Build Array("EnFlo Lab:labstrat1:Z=4.5m", "EnFlo Lab:labstrat1:Z=0.5m") -> (w693:string[])
          n238 = call "Read_Earlier_Channels.vi"("Present scan array"=w689, "Ch names"=w690, "Desired Channels"=w693) -> ("Scan comments"=w688:string, "Index 0"=w687:dbl, "Index 1"=w686:dbl)  [unwired: 3 out]
          n239 = Subtract(x=w687, y=w686) -> (x-y=w694:dbl)
        }
        frame "Laser:Cooling_Water:Delta_T" {
          n240 = Build Array("LDA Laser:Cooling water:Return Temp", "LDA Laser:Cooling water:Supply Temp") -> (w702:string[])
          n241 = call "Read_Earlier_Channels.vi"("Present scan array"=w698, "Ch names"=w699, "Desired Channels"=w702) -> ("Scan comments"=w697:string, "Index 0"=w696:dbl, "Index 1"=w695:dbl)  [unwired: 3 out]
          n242 = Subtract(x=w696, y=w695) -> (x-y=w703:dbl)
        }
        frame "EnFlo_Tunnel:Chilled Water:Valve Dem Pos" {
          n243 = Get Date/Time In Seconds() -> (seconds since 1Jan1904=w705:timestamp)
          n244 = Concatenate Strings(w706, " last updated") -> (w714:string)
          n245 = To Double Precision Float(number=w705) -> (double precision float=w704:dbl)
          n246 = Unbundle By Name(w712) -> ("A"=w711:dbl)
          n247 = call "Remember_value.vi"("Mode"=Remember_value_mode."Read only", "Ch name"=w714) -> ("Output Value"=w713:dbl)  [unwired: 1 in]
          n248 = Subtract(x=w704, y=w713) -> (x-y=w710:dbl)
          n249 = Greater?(x=w710, y=w711) -> (0:w709:bool)
          n250 = Not A Number/Path/Refnum?(number/path/refnum=w710) -> (NaN/Path/Refnum?=w708:bool)
          n251 = Or(x=w708, y=w709) -> (x .or. y?=w707:bool)
          n252 = case shown="True" w707 {
            tunnel: w721 -> [w722 w741]
            tunnel: [w722 w740] -> w720
            tunnel: w719 -> [_ w732]
            tunnel: w718 -> [_ w733]
            tunnel: ["" w738] -> w717
            tunnel: w714 -> [_ w728]
            tunnel: w704 -> [_ w724]
            frame False {
            }
            frame True {
              n253 = call "Read_value_of_earlier_Ch.vi"("Desired Ch to Read"="EnFlo_Tunnel:Chiller_Pump:Enable", "Ch names"=w733, "Present scan array"=w732) -> ("Value"=w731:dbl)  [unwired: 1 in, 1 out]
              n254 = Build Array("EnFlo_Tunnel:Chilled Water:Dem Temp", "EnFlo_Tunnel:Chilled Water:Supply", "EnFlo_Tunnel:Chiller_Pump:Running") -> (w739:string[])
              n255 = call "Read_Earlier_Channels.vi"("Present scan array"=w732, "Ch names"=w733, "Desired Channels"=w739) -> ("Scan comments"=w738:string, "Index 0"=w737:dbl, "Index 1"=w736:dbl, "Index 2"=w726:dbl)  [unwired: 2 out]
              n256 = Greater?(x=w731, y=0.5) -> (0:w729:bool)
              n257 = Greater?(x=w726, y=0.5) -> (0:w725:bool)
              n258 = case shown="False" w725 {
                tunnel: w741 -> [_ w769]
                tunnel: [w756 w763] -> w740
                tunnel: w737 -> [_ w765]
                tunnel: w736 -> [_ w764]
                tunnel: w724 -> [_ w762]
                tunnel: w729 -> [w747 _]
                tunnel: w728 -> [_ w761]
                frame False {
                  n259 = Seconds To Date/Time() -> (date time rec=w744:T13)  [unwired: 2 out]
                  n260 = Unbundle By Name(w744) -> ("day of week"=w751:i32, "hour"=w753:i32)
                  n261 = Less?(x=w753, y=3) -> (x < y?=w748:bool)
                  n262 = Equal?(x=7, y=w751) -> (x = y?=w749:bool)
                  n263 = And(x=w749, y=w748) -> (x .and. y?=w746:bool)
                  n264 = case shown="True" w747 {
                    tunnel: w746 -> [w757 w759]
                    tunnel: [w757 w758] -> w745
                    frame False {
                    }
                    frame True {
                      n265 = Not(x=w759) -> (.not. x?=w758:bool)
                    }
                  }
                  n266 = Select(t=0.0, s=w745, f=100.0) -> (s? t:f=w756:dbl)
                }
                frame True {
                  w767 = 100.0  # Max
                  w768 = 0.0  # Min
                  n267 = call "PID.vi"("Present Value"=w764, "Previous Control Sum"=w769, "Setpoint"=w765) -> ("Dem Output"=w766:dbl)
                  n268 = In Range and Coerce(upper limit=w767, x=w766, lower limit=w768) -> (coerced(x)=w763:dbl)  [unwired: 1 out]
                  n269 = call "Remember_value.vi"("Mode"=Remember_value_mode."Read and Write", "Input Value"=w762, "Ch name"=w761) -> ()  [unwired: 1 out]
                }
              }
            }
          }
        }
        frame "EnFlo_Tunnel:Hydrosonic:Integral" {
          n270 = Build Array("EnFlo_Tunnel:Usonic Fixed:Velocity", "Hydrosonic:Transducer:Setting") -> (w779:string[])
          n271 = call "Read_Earlier_Channels.vi"("Present scan array"=w780, "Ch names"=w778, "Desired Channels"=w779) -> ("Scan comments"=w772:string, "Index 0"=w777:dbl, "Index 1"=w771:dbl)  [unwired: 3 out]
          n272 = Greater?(x=w777, y=0.5) -> (0:w775:bool)
          n273 = case shown="True" w775 {
            tunnel: w774 -> [w783 w791]
            tunnel: [w783 w790] -> w773
            tunnel: w771 -> [_ w789]
            tunnel: w770 -> [_ w788]
            frame False {
            }
            frame True {
              w786 = 8640000.0  # Seconds per day x 100
              n274 = Multiply(x=w789, y=w788) -> (x*y=w787:dbl)
              n275 = Divide(x=w787, y=w786) -> (x/y=w785:dbl)
              n276 = Not A Number/Path/Refnum?(number/path/refnum=w785) -> (NaN/Path/Refnum?=w784:bool)
              n277 = case shown="False" w784 {
                tunnel: w791 -> [w794 w795]
                tunnel: [w793 w795] -> w790
                tunnel: w785 -> [w792 _]
                frame False {
                  n278 = Add(x=w792, y=w794) -> (x+y=w793:dbl)
                }
                frame True {
                }
              }
            }
          }
        }
        frame "EnFlo_Tunnel:Days Run at:2.5m/s" {
          n279 = Build Array("EnFlo_Tunnel:Usonic Fixed:Velocity") -> (w804:string[])
          n280 = call "Read_Earlier_Channels.vi"("Present scan array"=w805, "Ch names"=w803, "Desired Channels"=w804) -> ("Scan comments"=w798:string, "Index 0"=w796:dbl)  [unwired: 4 out]
          n281 = Greater?(x=w796, y=0.5) -> (0:w801:bool)
          n282 = case shown="True" w801 {
            tunnel: w800 -> [w807 w815]
            tunnel: [w807 w814] -> w799
            tunnel: w796 -> [_ w813]
            tunnel: w797 -> [_ w812]
            frame False {
            }
            frame True {
              w810 = 216000.0  # Seconds per day x 2.5
              n283 = Multiply(x=w813, y=w812) -> (x*y=w811:dbl)
              n284 = Divide(x=w811, y=w810) -> (x/y=w809:dbl)
              n285 = Not A Number/Path/Refnum?(number/path/refnum=w809) -> (NaN/Path/Refnum?=w808:bool)
              n286 = case shown="True" w808 {
                tunnel: w815 -> [w818 w819]
                tunnel: [w817 w819] -> w814
                tunnel: w809 -> [w816 _]
                frame False {
                  n287 = Add(x=w816, y=w818) -> (x+y=w817:dbl)
                }
                frame True {
                }
              }
            }
          }
        }
        frame "Complete:Scan:Period" {
          n288 = while {
            tunnel: [w829] -> w822
            tunnel: [w836] -> w824
            shift-left: _ -> [w836]
            shift-right: [w837] -> w825
            tunnel: w821 -> [w833]
            tunnel: [w828] -> w820
            stop <- FALSE continue-if-true
            w828 = 10.0 ("Averaging time (mins)")
            n289 = Build Array(w833) -> (w832:string[])
            n290 = call "Get_Channel_averages.vi"("Desired Ch Names"=w832, "Averaging time (mins)"=w828) -> ("number"=w831:dbl[])  [unwired: 1 in, 2 out]
            n291 = Index Array(array=w831, index=0) -> (element=w829:dbl)
            n292 = Greater?(x=w829, y=20.0) -> (0:w837:bool)
          }
          n293 = Compound Arithmetic op=AND(w825, invert w824) -> (w823:bool)
          n294 = case shown="True" w823 {
            tunnel: w822 -> [_ w843]
            tunnel: w820 -> [_ w838]
            frame False {
            }
            frame True {
              n295 = Format Into String(format string="Warning! The average scan period on the ADAM Scan table is %.1f seconds over the last %d minutes." ("Format String"), w843, w838) -> (resulting string=w841:string)  [unwired: 2 in, 1 out]
              n296 = call "Server_Emails.vi"("Message"=w841, "Contact All clients?"=TRUE, "Subject"="Scan Period") -> ()  [unwired: 2 in, 3 out]
            }
          }
        }
        frame "GMU:Source:Est Time" {
          # "NaN's"
          # "Est?"
          # "Inband?"
          n297 = stacked-sequence {
            seq-local: [w850 _ _ _] -> [_ _ w897 _]
            seq-local: [_ w862 _ _] -> [_ _ w894 _]
            seq-local: [_ w863 _ _] -> [_ _ w892 _]
            seq-local: [_ _ w899 _] -> [_ _ _ w915]
            seq-local: [w854 _ _ _] -> [_ _ w896 _]
            seq-local: [_ w861 _ _] -> [_ _ _ w911]
            tunnel: w849 -> [w856 w864 w902 _]
            tunnel: w848 -> [w855 w865 w903 _]
            tunnel: [_ _ w895 _] -> w847
            tunnel: [_ _ _ w914] -> w846
            tunnel: w845 -> [_ _ _ w913]
            tunnel: w844 -> [_ _ _ w912]
            frame #0 {
              n298 = Build Array("GMU:Source:Density Ratio", "GMU:Source:Dem Strength", "GMU:Source:Dem Q") -> (w857:string[])
              n299 = call "Read_Earlier_Channels.vi"("Present scan array"=w855, "Ch names"=w856, "Desired Channels"=w857) -> ("Scan comments"=w854:string, "Index 0"=w853:dbl, "Index 1"=w852:dbl, "Index 2"=w851:dbl)  [unwired: 2 out]
              n300 = Build Array(w853, w852, w851) -> (w850:dbl[])
            }
            frame #1 {
              n301 = for {
                N: 2 -> [_]
                tunnel: w865 -> [w875]
                tunnel: w864 -> [w876]
                tunnel: [w874] -> w862 mode=indexing
                tunnel: [w881] -> w863 mode=indexing
                tunnel: [w880] -> w861 mode=indexing
                i -> [w886]
                w885 = 23.0  # %
                n302 = case shown="1" w886 {
                  tunnel: ["GMU:Source:Meas Q" "GMU:Source:Meas Strength"] -> w879
                  tunnel: ["GMU:Source:Dem Q" "GMU:Source:Dem Strength"] -> w878
                  frame 0, Default {
                  }
                  frame 1 {
                  }
                }
                n303 = Build Array(w878, w879) -> (w877:string[])
                n304 = call "Read_Earlier_Channels.vi"("Present scan array"=w875, "Ch names"=w876, "Desired Channels"=w877) -> ("Scan comments"=w874:string, "Index 0"=w872:dbl, "Index 1"=w873:dbl)  [unwired: 3 out]
                n305 = Not A Number/Path/Refnum?(number/path/refnum=w873) -> (NaN/Path/Refnum?=w880:bool)
                n306 = Subtract(x=w873, y=w872) -> (x-y=w871:dbl)
                n307 = Greater Than 0?(x=w872) -> (x > 0?=w882:bool)
                n308 = Less?(x=w871, y=0.05) -> (x < y?=w868:bool)
                n309 = call "In_Range_check.vi"("%"=w885, "Mode"=In_Range."%", "Value"=w873, "Setpoint"=w872) -> ("In Range"=w869:bool)  [unwired: 1 in, 2 out]
                n310 = Or(x=w869, y=w868) -> (x .or. y?=w867:bool)
                n311 = And(x=w867, y=w882) -> (x .and. y?=w883:bool)
                n312 = Compound Arithmetic op=OR(w883, invert w882, w880) -> (w881:bool)
              }
            }
            frame #2 {
              n313 = while {
                tunnel: [w910] -> w898
                tunnel: w897 -> [w909]
                shift-left: _ -> [w910]
                shift-right: [w909] -> _
                stop <- FALSE continue-if-true
              }
              n314 = Equal?(x=w897, y=w898) -> (x = y?=w904:bool)
              n315 = call "Read_value_of_earlier_Ch.vi"("Desired Ch to Read"="GMU:Source:Dem Q", "Ch names"=w902, "Present scan array"=w903) -> ("Value"=w900:dbl)  [unwired: 1 in, 1 out]
              n316 = Greater Than 0?(x=w900) -> (x > 0?=w907:bool)
              n317 = And Array Elements(Boolean array=w892) -> (logical AND=w891:bool)
              n318 = Select(t=w891, s=w907, f=TRUE) -> (s? t:f=w905:bool)
              n319 = Compound Arithmetic op=AND(w904, w905) -> (w899:bool)
              n320 = Concatenate Strings(w894) -> (w893:string)
              n321 = Concatenate Strings(w893, w896) -> (w895:string)
            }
            frame #3 {
              n322 = case shown="True" w915 {
                tunnel: [0.0 w917] -> w914
                tunnel: w913 -> [_ w922]
                tunnel: w912 -> [_ w918]
                tunnel: w911 -> [_ w921]
                frame False {
                }
                frame True {
                  n323 = Or Array Elements(Boolean array=w921) -> (logical OR=w920:bool)
                  n324 = Add(x=w922, y=w918) -> (x+y=w919:dbl)
                  n325 = Select(t=w918, s=w920, f=w919) -> (s? t:f=w917:dbl)
                }
              }
            }
          }
        }
      }
    }
    frame "Hold Value" {
    }
    frame "Read A" {
      n326 = Unbundle By Name(w926) -> ("A"=w925:dbl)
    }
    frame "Read Ch" {
      n327 = Unbundle By Name(w931) -> ("String"=w928:string)
      n328 = call "Read_value_of_earlier_Ch.vi"("Desired Ch to Read"=w928, "Ch names"=w932, "Present scan array"=w933) -> ("Value"=w929:dbl, "Scan comment"=w930:string)  [unwired: 1 in]
    }
    frame "Coded" {
    }
    frame "Client Info" {
      n329 = global read "ADAM_Global.vi" "Client State Array"() -> (w948:T14[])
      n330 = call "Split_Ch_name.vi"("Ch name"=w942) -> ("Top level"=w940:string, "Low level"=w938:string)  [unwired: 1 out]
      n331 = Equal?(x="Status" ("Substring"), y=w940) -> (x = y?=w939:bool)
      n332 = Select(t=w938, s=w939, f="") -> (s? t:f=w936:string)
      n333 = for {
        tunnel: w948 -> [w957] mode=indexing
        tunnel: [w956] -> w949 mode=indexing
        n334 = Unbundle By Name(w957) -> ("Client Name"=w956:string)
      }
      n335 = Search 1D Array(1D array=w949, element=w936) -> (index of element=w944:i32)  [unwired: 1 out]
      n336 = Less Than 0?(x=w944) -> (x < 0?=w943:bool)
      n337 = Index Array(array=w948, index=w944) -> (element=w947:T14)
      n338 = case shown="False" w943 {
        tunnel: w947 -> [w952 _]
        tunnel: w936 -> [w951 w954]
        tunnel: [w950 w953] -> w946
        frame False {
          n339 = call "Get_Client_Status_string.vi"("Client State Cluster"=w952, "Client Name"=w951) -> ("Code Value"=w950:dbl)  [unwired: 1 in]
        }
        frame True {
          w953 = 7.0 ("Code Value")
          n340 = call "Remember_value.vi"("Mode"=Remember_value_mode."Read and Write", "Input Value"=w953, "Ch name"=w954) -> ()  [unwired: 1 out]
        }
      }
    }
    frame "Web Client" {
      w967 = 7200.0  # 2 Hours in Seconds
      n341 = Concatenate Strings(w976, ":Last read" ("Substring")) -> (w974:string)
      n342 = call "Remember_value.vi"("Mode"=Remember_value_mode."Read only", "Ch name"=w974) -> ("Output Value"=w973:dbl)  [unwired: 1 in]
      n343 = Not A Number/Path/Refnum?(number/path/refnum=w973) -> (NaN/Path/Refnum?=w971:bool)
      n344 = Get Date/Time In Seconds() -> (seconds since 1Jan1904=w966:timestamp)
      n345 = To Double Precision Float(number=w966) -> (double precision float=w964:dbl)
      n346 = Subtract(x=w964, y=w973) -> (x-y=w979:dbl)
      n347 = Greater?(x=w979, y=1800.0) -> (0:w972:bool)
      n348 = Or(x=w972, y=w971) -> (x .or. y?=w958:bool)
      n349 = case shown="True" w958 {
        frame False {
        }
        frame True {
          n350 = global read "Constants_global.vi" "EnFlo SW Folder"() -> (w982:path)
          n351 = Build Path(base path=w982, name or relative path=path "ADAM Server/Sub VI's/Web_Client.vi") -> (appended path=w981:path)
          n352 = Open VI Reference(vi path=w981) -> (vi reference=w986:refnum<vi>, error out=w987:errorcluster)  [unwired: 1 in, 4 out]
          n353 = property class="VI"(reference=w986, error in=w987) -> (reference out=w989:refnum<vi>, error out=w990:errorcluster, "Front Panel Window:Open"=w988:bool)
          n354 = case shown="False" w988 {
            tunnel: w989 -> [w996 w999]
            tunnel: w990 -> [w995 w998]
            tunnel: [w994 w999] -> w991
            tunnel: [w993 w998] -> w992
            frame False {
              n355 = property class="VI"(reference=w996, error in=w995, "Front Panel Window:Open"=TRUE) -> (reference out=w994:refnum<vi>, error out=w993:errorcluster)
            }
            frame True {
            }
          }
          n356 = invoke class="VI" method="Run VI"(reference=w991, error in=w992, "Wait until done"=FALSE, "Auto Dispose Ref"=TRUE) -> ()  [unwired: 1 in, 5 out]
        }
      }
      n357 = Concatenate Strings(w976, ":value time" ("Substring")) -> (w960:string)
      n358 = call "Remember_value.vi"("Mode"=Remember_value_mode."Read only", "Ch name"=w976) -> ("Output Value"=w980:dbl)  [unwired: 1 in]
      n359 = call "Remember_value.vi"("Mode"=Remember_value_mode."Read only", "Ch name"=w960) -> ("Output Value"=w965:dbl)  [unwired: 1 in]
      n360 = Subtract(x=w964, y=w965) -> (x-y=w963:dbl)
      n361 = Greater?(x=w963, y=w967) -> (0:w970:bool)
      n362 = case shown="True" w970 {
        tunnel: w963 -> [_ w1005]
        tunnel: 3600.0 ("y") -> [_ w1004]
        tunnel: ["" w1002] -> w969
        frame False {
        }
        frame True {
          n363 = Divide(x=w1005, y=w1004) -> (x/y=w1001:dbl)
          n364 = Format Into String(format string="Value is %d hours old." ("Format String"), w1001) -> (resulting string=w1002:string)  [unwired: 2 in, 1 out]
        }
      }
    }
    frame "X10" {
      (unwired) 1 items=["-----", "A", "B", "C", "D", "E", "F", "G", "H", "I", "J", "K", "L", "M", "N", "O", "P"] ("House Code")
      n365 = Greater Than 0?(x=w1010) -> (x > 0?=w1009:bool)
      n366 = Unbundle By Name(w1015) -> ("Port Name"=w1012:string, "Main"=w1013:i32, "Ch."=w1014:i32)
      n367 = call "X10control.vi"("Port Name"=w1012, "Power Request (ON)"=w1009, "House Code"=w1013, "Unit No."=w1014) -> ()  [unwired: 6 out]
      n368 = Select(t=1.0, s=w1009, f=0.0) -> (s? t:f=w1006:dbl)
    }
    frame "LPA" {
      # "LPA was, IIRC, a serially-polled weighing platform we rented at Surrey for Athena Scaperdas' project at Atkins to weigh a helicopter with rotor running. \nTo add to the fun, it was RS232, so to make it addressable it was polled through an addressable ADAM 485-232 module"
      n369 = call "LPA400_get_rdg.vi"("Channel Name"=w1018, "Address"=w1019) -> ("Output"=w1016:dbl, "Status note"=w1017:string)  [unwired: 4 out]
    }
    frame "ScanPacer" {
      # "Uses a metronome to slow an otherwise over-fast scan table"
      n370 = call "ADAMPacer.vi"("Ch Description"=w1022) -> ("Scan comment"=w1020:string, "Output"=w1021:dbl)  [unwired: 7 in]
    }
    frame "Test" {
      w1026 = 0.0005  # y
      n371 = Get Date/Time In Seconds() -> (seconds since 1Jan1904=w1023:timestamp)
      n372 = To Double Precision Float(number=w1023) -> (double precision float=w1028:dbl)
      n373 = Subtract(x=w1028, y=2969882881.0) -> (x-y=w1027:dbl)
      n374 = Multiply(x=w1027, y=w1026) -> (x*y=w1024:dbl)
      n375 = Random Number (0-1)() -> (number: 0 to 1=w1025:dbl)
      n376 = Add(x=w1025, y=w1024) -> (x+y=w1031:dbl)
    }
    frame "Oops", Default {
    }
  }
  "Output" <- w8
  "Scan comment" <- w5
